vi "Check Idle.vi"(8 "error in (no error)":errorcluster, 10 "Controller #":string, 11 "Port In":T1={"P type"=0, "reference"="", " Terminator "="\r\n", "Timeout"=300} {"Timeout" step=10; "P type" items=["none", "RS-232C"]}) -> (0 "error out (no error)":errorcluster, 3 "Port Out":T1)   [LabVIEW 2021]
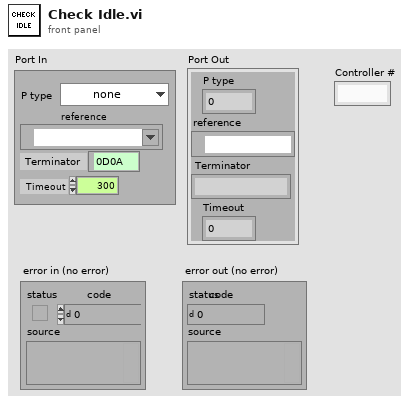
[diagram p1: front panel]
types:
  T1 = cluster{"P type":u16, "reference":refnum<visa-resource-name>, " Terminator ":string, "Timeout":i32}
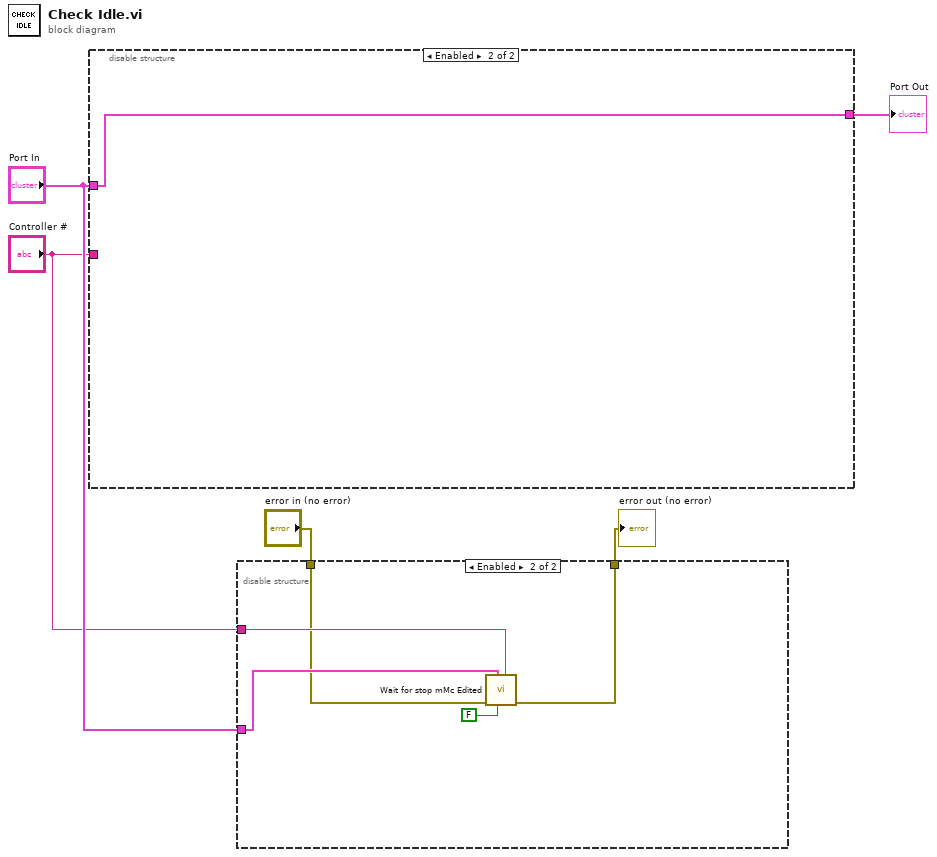
[diagram p0: block diagram]
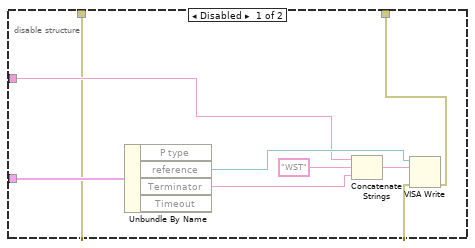
[diagram p2: hidden frame]
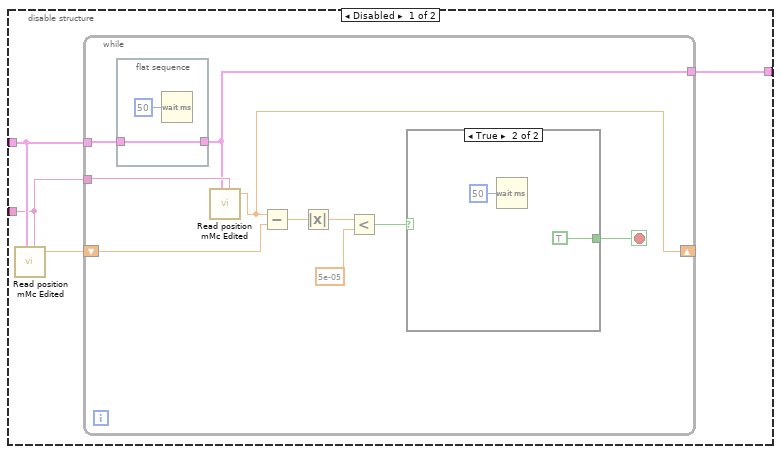
[diagram p3: hidden frame]
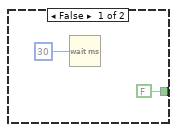
[diagram p4: hidden frame]
diagram:
  n1 = disable-structure shown="Enabled" {
    disable-tunnel: [w8 w26] -> w5
    disable-tunnel: "Port In" -> [w7 w26]
    disable-tunnel: "Controller #" -> [w6 _]
    frame Disabled {
      n2 = call "Read position mMc Edited.vi"("Port"=w7, "Controller #"=w6) -> ("Cnt pos"=w9:dbl)  [unwired: 5 in, 2 out]
      n3 = while {
        tunnel: w7 -> [w13]
        shift-right: [w11] -> _
        shift-left: w9 -> [w19]
        tunnel: w6 -> [w12]
        tunnel: [w10] -> w8
        stop <- w14 stop-if-true
        n4 = flat-sequence {
          tunnel: [w21] -> w10
          tunnel: w13 -> [w21]
          frame #0 {
            n5 = Wait (ms)(milliseconds to wait=u32 50) -> ()  [unwired: 1 out]
          }
        }
        n6 = call "Read position mMc Edited.vi"("Port"=w10, "Controller #"=w12) -> ("Cnt pos"=w11:dbl)  [unwired: 5 in, 2 out]
        n7 = Subtract(x=w11, y=w19) -> (x-y=w17:dbl)
        n8 = Absolute Value(x=w17) -> (abs(x)=w16:dbl)
        n9 = Less?(x=w16, y=5e-05) -> (x < y?=w15:bool)
        n10 = case shown="True" w15 {
          tunnel: [FALSE TRUE] -> w14
          frame False {
            n11 = Wait (ms)(milliseconds to wait=u32 30) -> ()  [unwired: 1 out]
          }
          frame True {
            n12 = Wait (ms)(milliseconds to wait=u32 50) -> ()  [unwired: 1 out]
          }
        }
      }
    }
    frame Enabled {
    }
  }
  "Port Out" <- w5
  n13 = disable-structure shown="Enabled" {
    disable-tunnel: "Port In" -> [w31 w38]
    disable-tunnel: "Controller #" -> [w30 w39]
    disable-tunnel: "error in (no error)" -> [w28 w35]
    disable-tunnel: [w27 w36] -> w2
    frame Disabled {
      n14 = Unbundle By Name(w31) -> ("reference"=w32:refnum<visa-resource-name>, "Terminator"=w33:string)  [unwired: 2 out]
      n15 = Concatenate Strings(w30, "WST" ("string"), w33) -> (w34:string)
      n16 = VISA Write(VISA resource name=w32, write buffer=w34, error in (no error)=w28) -> (error out=w27:errorcluster)  [unwired: 2 out]
    }
    frame Enabled {
      n17 = call "Wait for stop mMc Edited.vi"("Controller #"=w39, "wait for in pos"=FALSE, "Port"=w38, "error in (no error)"=w35) -> ("error out"=w36:errorcluster)  [unwired: 7 in]
    }
  }
  "error out (no error)" <- w2
